vi "Autonomous Independent.vi"() -> ()   [LabVIEW 2017]
doc: "This VI is called when autonomous begins, and will automatically be terminated when autonomous ends. You can carry out timed or sensor driven robot movement independently without needing to return to the caller."
uses:
  <vilib>/Rock Robotics/WPI/Utilities/WPI_GetSetVariantRefNum.vi
  <vilib>/Rock Robotics/Network Tables/NT Read String.vi
  <vilib>/Rock Robotics/Network Tables/NT Read Number.vi
  <vilib>/Rock Robotics/Network Tables/NT Read Boolean.vi
  <vilib>/Rock Robotics/WPI/RobotDrive/WPI_RobotDriveArcadeDrive_Standard(NoSaturation).vi
  <vilib>/Rock Robotics/Network Tables/NT Write Numeric Array.vi
panel:
  in  "1 switch":T1(array[cluster])=[{"Movement"="Pause", "Delay (sec)"=1.0, "X Joystick Value"=0.0, "Y Joystick Value"=0.0}, {"Movement"="Forward 90 in", "Delay (sec)"=4.5, "X Joystick Value"=0.0, "Y Joystick Value"=0.5}, {"Movement"="Puase", "Delay (sec)"=1.0, "X Joystick Value"=0.0, "Y Joystick Value"=0.0}, {"Movement"="Slow Turn 90", "Delay (sec)"=0.55, "X Joystick Value"=0.7, "Y Joystick Value"=0.0}, {"Movement"="Pause", "Delay (sec)"=1.0, "X Joystick Value"=0.0, "Y Joystick Value"=0.0}, {"Movement"="Jolt", "Delay (sec)"=0.3, "X Joystick Value"=0.0, "Y Joystick Value"=1.0}, {"Movement"="Pause", "Delay (sec)"=1.0, "X Joystick Value"=0.0, "Y Joystick Value"=0.0}]
  in  "3 Switch":T1(array[cluster])=[{"Movement"="Pause", "Delay (sec)"=1.0, "X Joystick Value"=0.0, "Y Joystick Value"=0.0}, {"Movement"="Forward 90 in", "Delay (sec)"=4.5, "X Joystick Value"=0.0, "Y Joystick Value"=0.5}, {"Movement"="Puase", "Delay (sec)"=1.0, "X Joystick Value"=0.0, "Y Joystick Value"=0.0}, {"Movement"="slow turn 90", "Delay (sec)"=0.55, "X Joystick Value"=-0.7, "Y Joystick Value"=0.0}, {"Movement"="Pause", "Delay (sec)"=1.0, "X Joystick Value"=0.0, "Y Joystick Value"=0.0}, {"Movement"="Jolt", "Delay (sec)"=0.3, "X Joystick Value"=0.0, "Y Joystick Value"=1.0}, {"Movement"="Pause", "Delay (sec)"=1.0, "X Joystick Value"=0.0, "Y Joystick Value"=0.0}]
  in  "2 line 2":T1(array[cluster])=[{"Movement"="Pause", "Delay (sec)"=1.0, "X Joystick Value"=0.0, "Y Joystick Value"=0.0}, {"Movement"="Forward 90 in", "Delay (sec)"=4.5, "X Joystick Value"=0.0, "Y Joystick Value"=0.5}, {"Movement"="Puase", "Delay (sec)"=1.0, "X Joystick Value"=0.0, "Y Joystick Value"=0.0}, {"Movement"="Forward 60\nForward 60 in", "Delay (sec)"=1.0, "X Joystick Value"=0.0, "Y Joystick Value"=0.0}, {"Movement"="Forward 90 in", "Delay (sec)"=1.0, "X Joystick Value"=0.0, "Y Joystick Value"=0.0}, {"Movement"="Forward 90 in", "Delay (sec)"=1.0, "X Joystick Value"=0.0, "Y Joystick Value"=0.0}]
  in  "2 line 1":T1(array[cluster])=[{"Movement"="Pause", "Delay (sec)"=1.0, "X Joystick Value"=0.0, "Y Joystick Value"=0.0}, {"Movement"="Forward 90 in", "Delay (sec)"=4.5, "X Joystick Value"=0.0, "Y Joystick Value"=0.5}, {"Movement"="Puase", "Delay (sec)"=1.0, "X Joystick Value"=0.0, "Y Joystick Value"=0.0}, {"Movement"="Pause\nForward 60 in", "Delay (sec)"=1.0, "X Joystick Value"=0.0, "Y Joystick Value"=0.0}, {"Movement"="Pause", "Delay (sec)"=1.0, "X Joystick Value"=0.0, "Y Joystick Value"=0.0}, {"Movement"="Pause", "Delay (sec)"=1.0, "X Joystick Value"=0.0, "Y Joystick Value"=0.0}]
  in  "3 line":T1(array[cluster])=[{"Movement"="Pause", "Delay (sec)"=0.0, "X Joystick Value"=0.0, "Y Joystick Value"=0.0}, {"Movement"="Forward 90 in", "Delay (sec)"=4.5, "X Joystick Value"=0.0, "Y Joystick Value"=0.5}, {"Movement"="Puase", "Delay (sec)"=1.0, "X Joystick Value"=0.0, "Y Joystick Value"=0.0}, {"Movement"="Back ", "Delay (sec)"=1.0, "X Joystick Value"=0.0, "Y Joystick Value"=0.0}, {"Movement"="Forward 90 in", "Delay (sec)"=1.0, "X Joystick Value"=0.0, "Y Joystick Value"=0.0}, {"Movement"="Forward 90 in", "Delay (sec)"=1.0, "X Joystick Value"=0.0, "Y Joystick Value"=0.0}]
  in  "1 Line":T1(array[cluster])=[{"Movement"="Pause", "Delay (sec)"=1.0, "X Joystick Value"=0.0, "Y Joystick Value"=0.0}, {"Movement"="Forward 90 in", "Delay (sec)"=4.5, "X Joystick Value"=0.0, "Y Joystick Value"=0.5}, {"Movement"="Puase", "Delay (sec)"=1.0, "X Joystick Value"=0.0, "Y Joystick Value"=0.0}, {"Movement"="back 60\nForward 60 in", "Delay (sec)"=1.0, "X Joystick Value"=0.0, "Y Joystick Value"=0.0}, {"Movement"="Forward 90 in", "Delay (sec)"=1.0, "X Joystick Value"=0.0, "Y Joystick Value"=0.0}, {"Movement"="Forward 90 in", "Delay (sec)"=1.0, "X Joystick Value"=0.0, "Y Joystick Value"=0.0}]
  in  "Auto Main 2":T1(array[cluster])=[{"Movement"="Pause", "Delay (sec)"=1.0, "X Joystick Value"=0.0, "Y Joystick Value"=0.0}, {"Movement"="Forward 90 in", "Delay (sec)"=2.2, "X Joystick Value"=0.0, "Y Joystick Value"=0.7}, {"Movement"="Puase", "Delay (sec)"=1.0, "X Joystick Value"=0.0, "Y Joystick Value"=0.0}, {"Movement"="Forward 60\nForward 60 in", "Delay (sec)"=1.0, "X Joystick Value"=0.0, "Y Joystick Value"=0.0}, {"Movement"="Forward 90 in", "Delay (sec)"=1.0, "X Joystick Value"=0.0, "Y Joystick Value"=0.0}, {"Movement"="Forward 90 in", "Delay (sec)"=1.0, "X Joystick Value"=0.0, "Y Joystick Value"=0.0}]
  out "Current Movement, for debugging":T2 {"Y Joystick Value" scale=1.0..-1.0; "X Joystick Value" scale=-1.0..1.0}
  in  "Array of robot movements":T3(array[cluster])=[{"X Joystick Value"=0.39393939393939403, "Y Joystick Value"=0.0, "Delay (sec)"=1.0, "Movement Name"="turn"}, {"X Joystick Value"=-0.3737373737373737, "Y Joystick Value"=0.0, "Delay (sec)"=1.0, "Movement Name"="turn back"}] {"Y Joystick Value" scale=1.0..-1.0; "X Joystick Value" scale=-1.0..1.0}
  # "Be sure to right-click and choose Data Operations>>Make Current Value default if you want to save the array values with the VI"
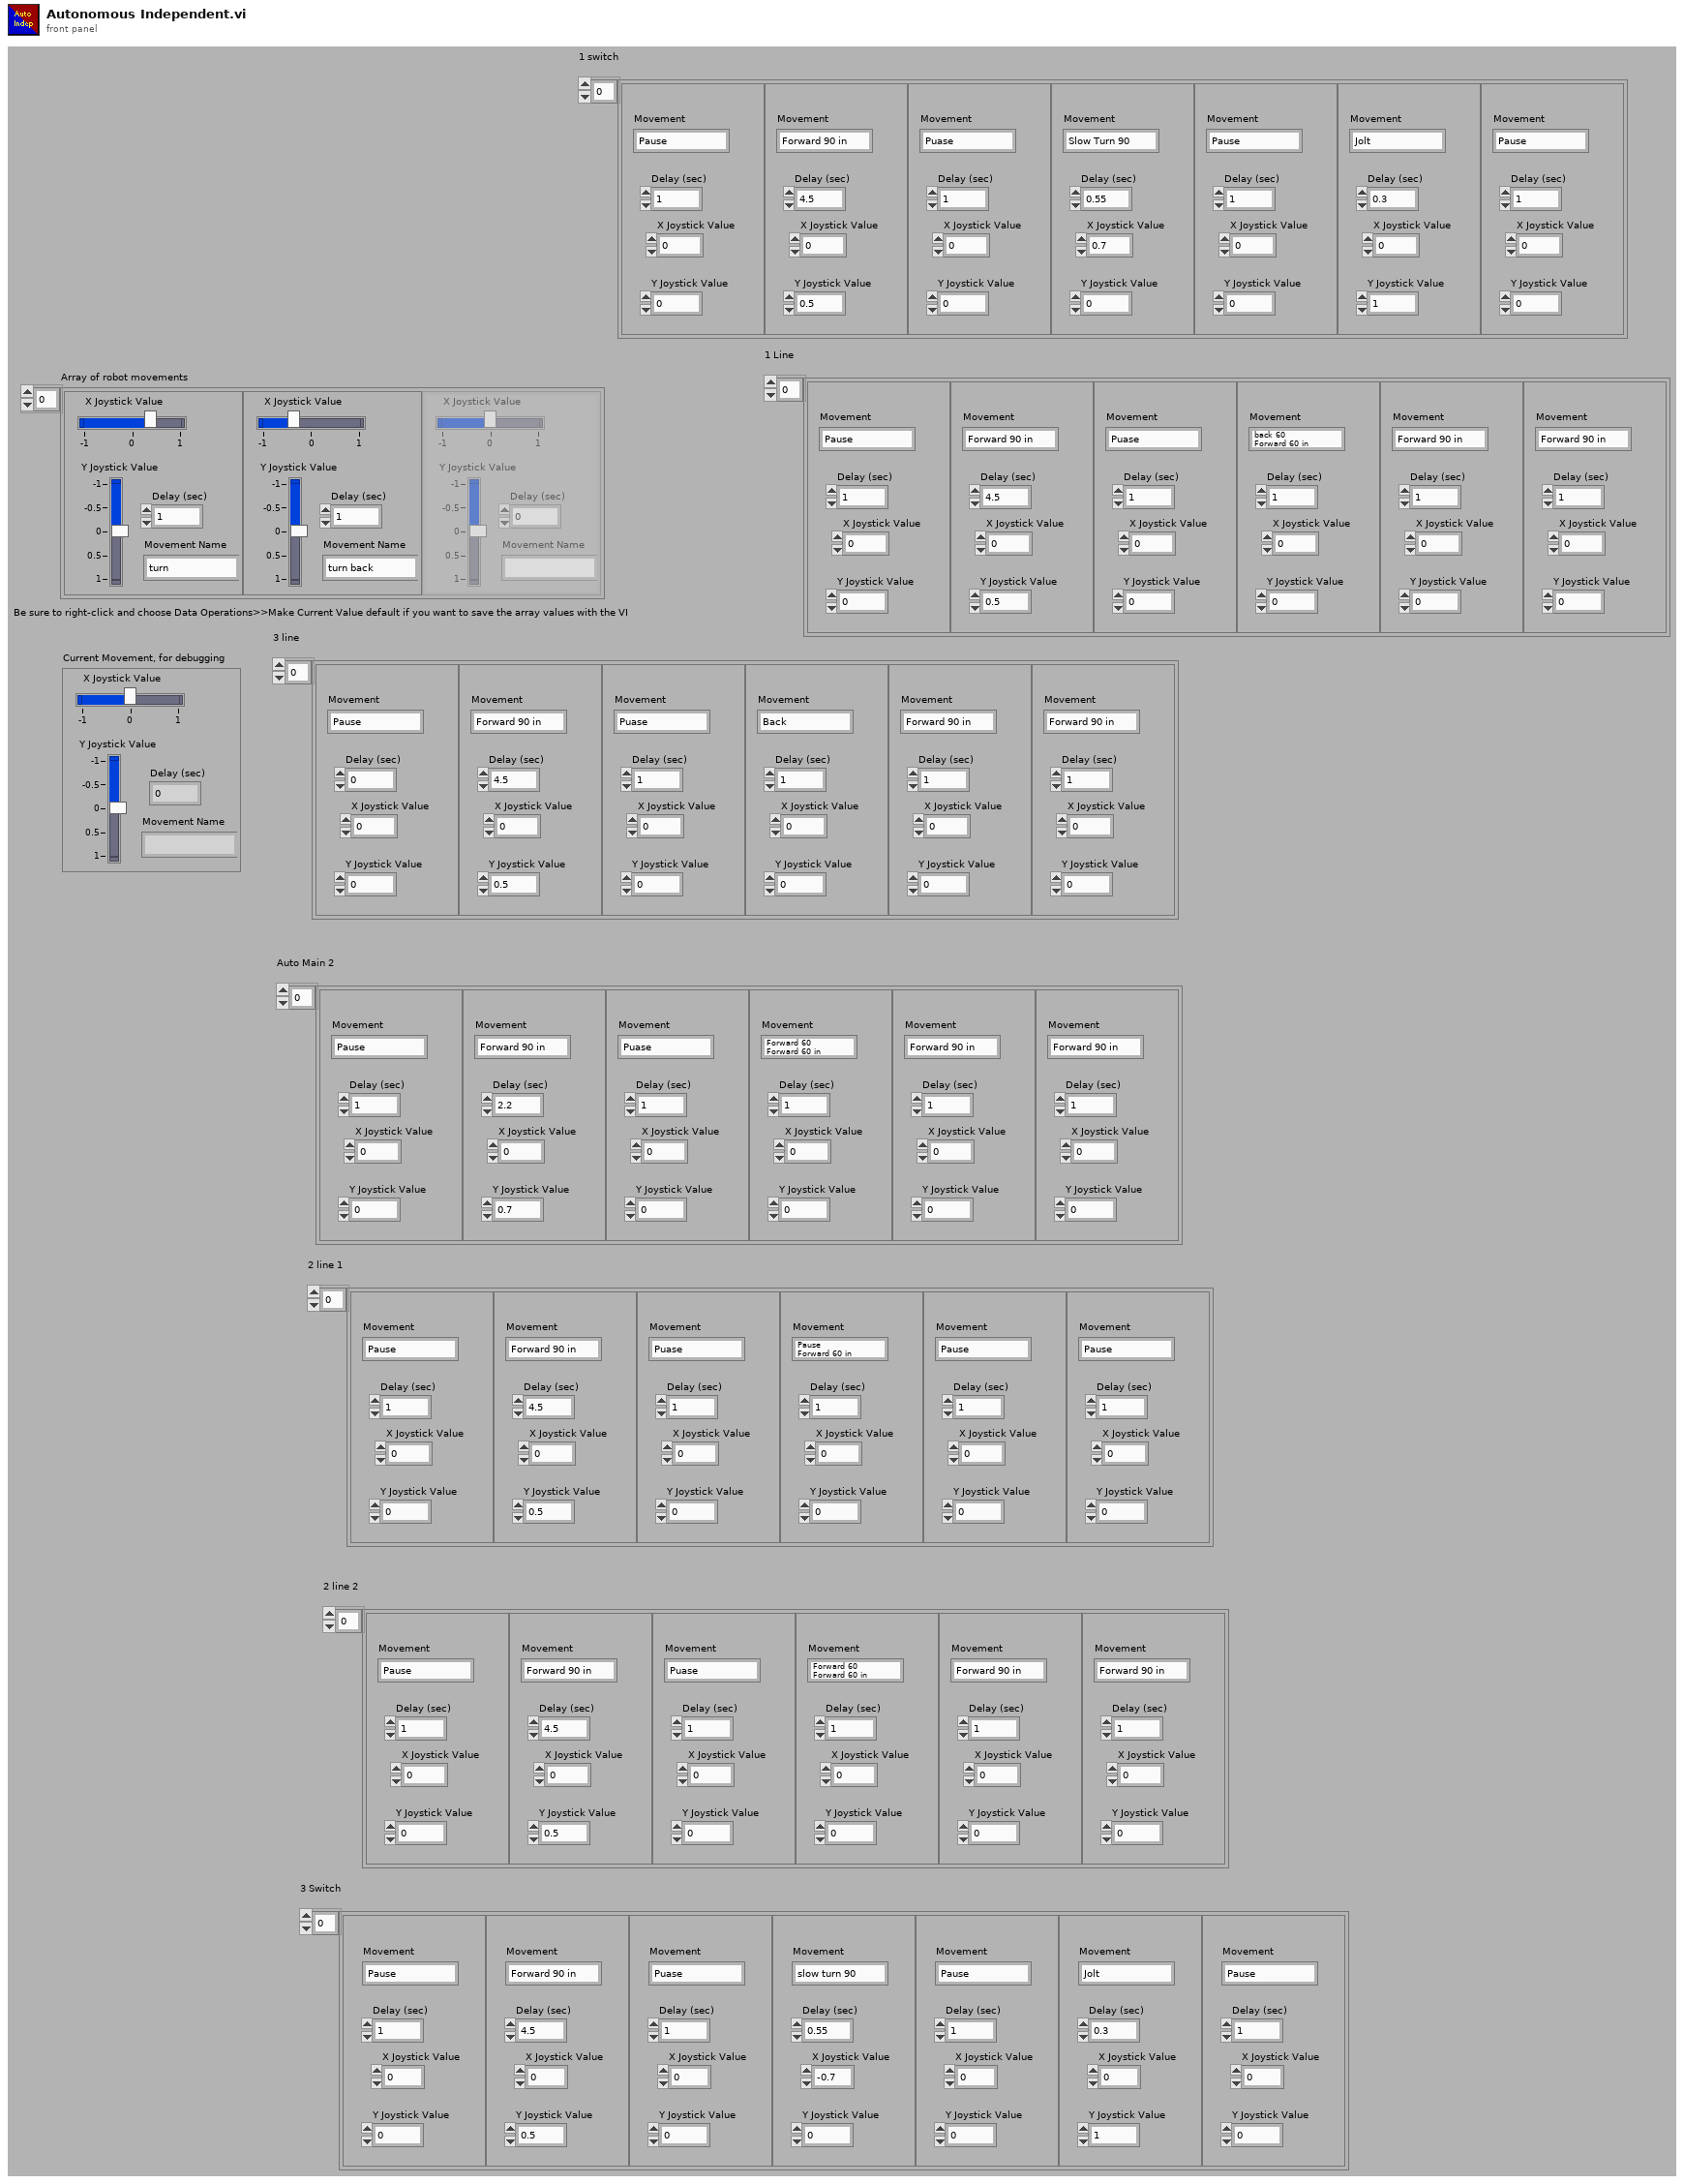
[diagram p1: front panel]
types:
  T1 = cluster{"Movement":string, "Delay (sec)":dbl, "X Joystick Value":dbl, "Y Joystick Value":dbl}[]
  T2 = cluster{"X Joystick Value":dbl, "Y Joystick Value":dbl, "Delay (sec)":dbl, "Movement Name":string}
  T3 = cluster{"X Joystick Value":dbl, "Y Joystick Value":dbl, "Delay (sec)":dbl, "Movement Name":string}[]
  T4 = typedef "WPI_JoystickDevRef.ctl" = cluster{"Device":T5}
  T5 = typedef "WPI_JoystickDeviceEnum.ctl" = enum16{"USB 0", "USB 1", "USB 2", "USB 3", "USB 4", "USB 5"}
  T6 = typedef "WPI_RobotDriveDevRef.ctl" = cluster{"DevStatus":errorcluster, "Motors[]":T7[], "Square Inputs":bool, "Max Output":dbl}
  T7 = typedef "WPI_MotorControlDeviceRef.ctl" = cluster{"DeviceStatus":errorcluster, "Type":T8, "PWM":cluster{"PWM Channel":T9, "DeadBand":T10}, "CAN":cluster{"Device Number":u8, "SetOutput VI Ref":variant, "GetOutput VI Ref":variant, "Enable VI Ref":variant, "Disable VI Ref":variant, "Data":variant}, "Invert":bool, "DIO PWM":cluster{"PWM \"Enable\" Channel":T9, "DIOChannel":T11, "PWM Rate":dbl}}
  T8 = typedef "WPI_MotorControlType.ctl" = enum16{"PWM", "CAN", "DIO PWM"}
  T9 = typedef "FPGA_DIOPWMChannel.ctl" = enum8{"PWM 0", "PWM 1", "PWM 2", "PWM 3", "PWM 4", "PWM 5", "PWM 6", "PWM 7", "PWM 8", "PWM 9", "PWM MXP 0", "PWM MXP 1", "PWM MXP 2", "PWM MXP 3", "PWM MXP 4", "PWM MXP 5", "PWM MXP 6", "PWM MXP 7", "PWM MXP 8", "PWM MXP 9", "Invalid"}
  T10 = typedef "WPI_PWMDeadband.ctl" = cluster{"Name":string, "maxPositivePwm":i32, "minPositivePwm":i32, "centerPwm":i32, "maxNegativePwm":i32, "minNegativePwm":i32, "angularRange":u16}
  T11 = typedef "FPGA_DIOChannel.ctl" = enum8{"DIO 0", "DIO 1", "DIO 2", "DIO 3", "DIO 4", "DIO 5", "DIO 6", "DIO 7", "DIO 8", "DIO 9", "DIO MXP 0", "DIO MXP 1", "DIO MXP 2", "DIO MXP 3", "DIO MXP 4", "DIO MXP 5", "DIO MXP 6", "DIO MXP 7", "DIO MXP 8", "DIO MXP 9", "DIO MXP 10", "DIO MXP 11", "DIO MXP 12", "DIO MXP 13", "DIO MXP 14", "DIO MXP 15", "SPI Port CS1", "SPI Port CS2", "SPI Port CS3", "SPI Port MISO", "SPI Port MOSI", "Invalid"}
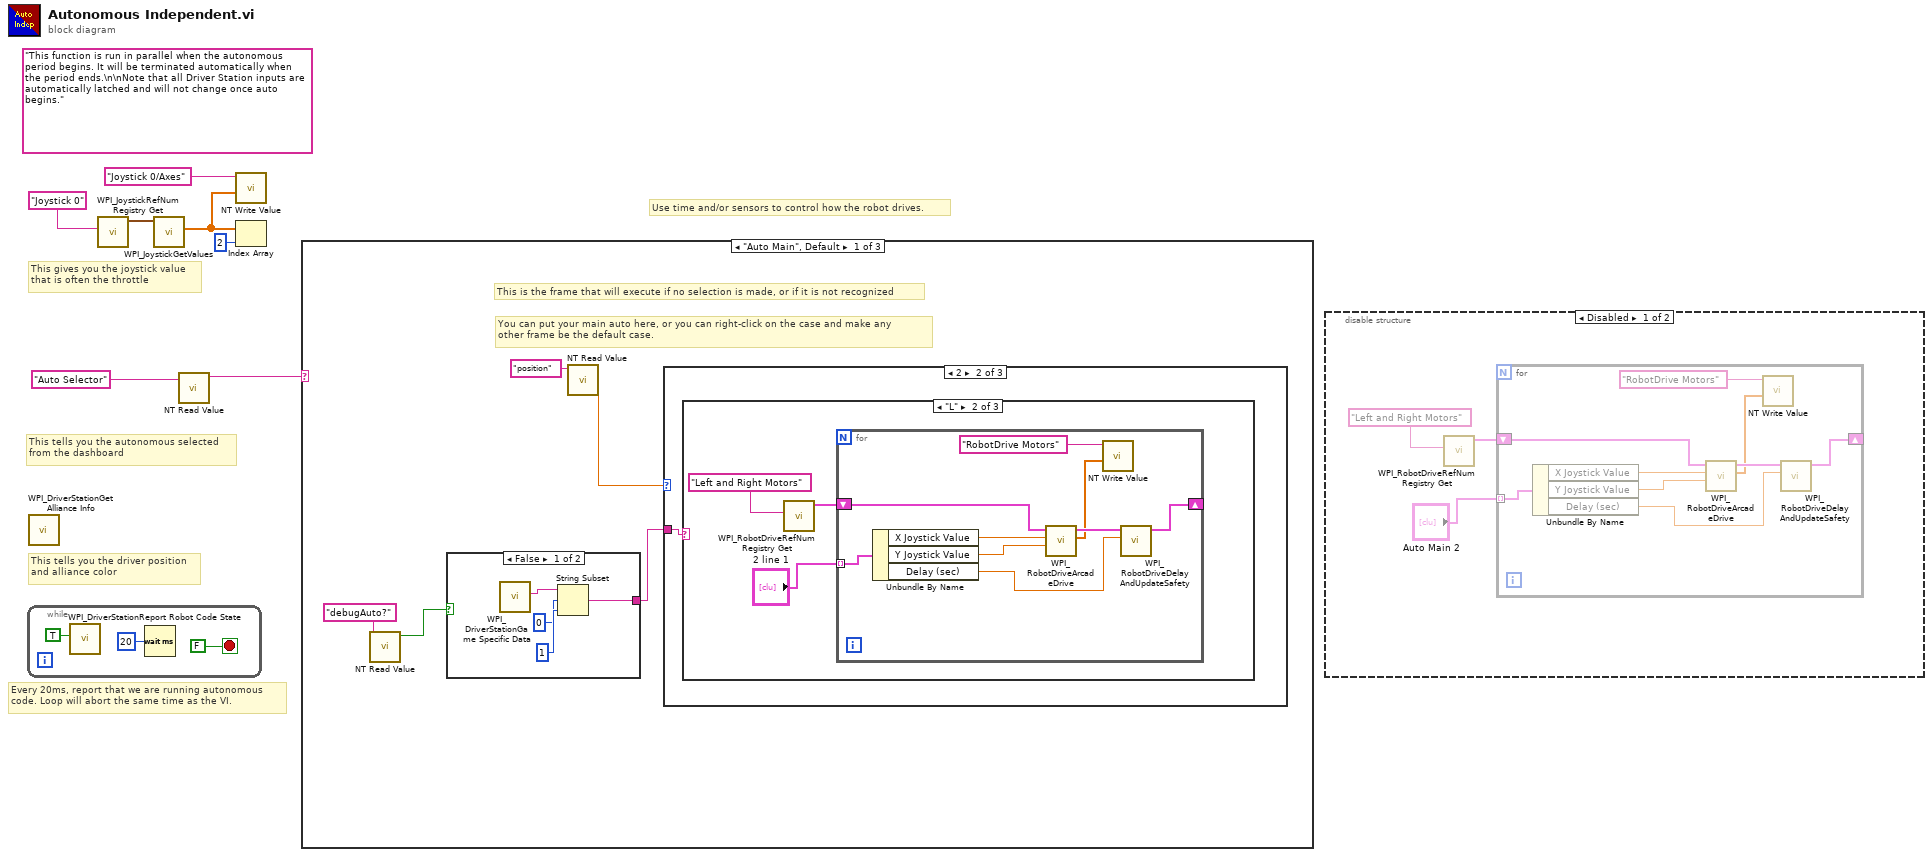
[diagram p0: block diagram]
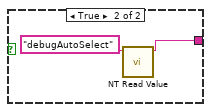
[diagram p3: hidden frame]
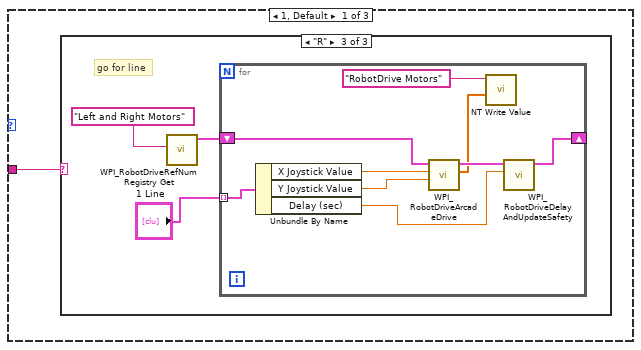
[diagram p4: hidden frame]
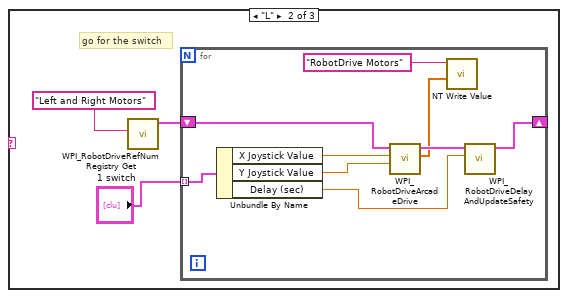
[diagram p6: hidden frame]
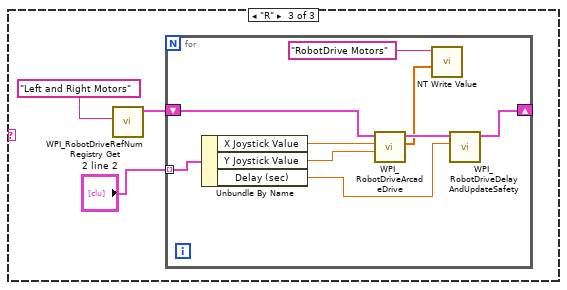
[diagram p8: hidden frame]
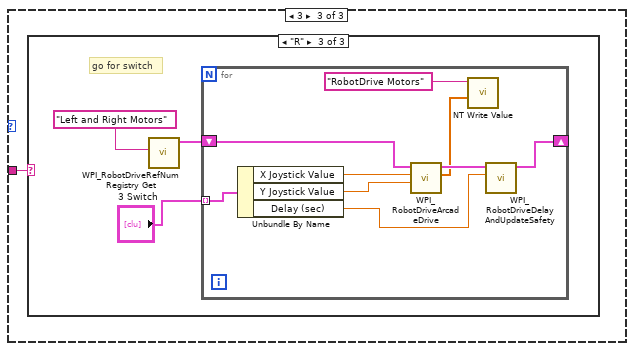
[diagram p9: hidden frame]
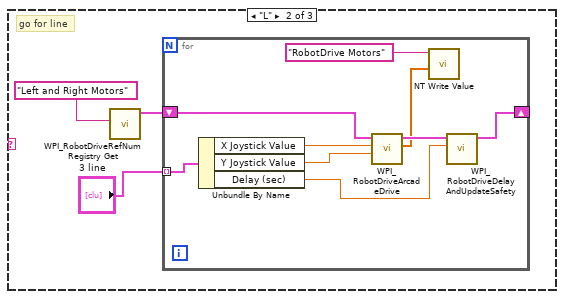
[diagram p11: hidden frame]
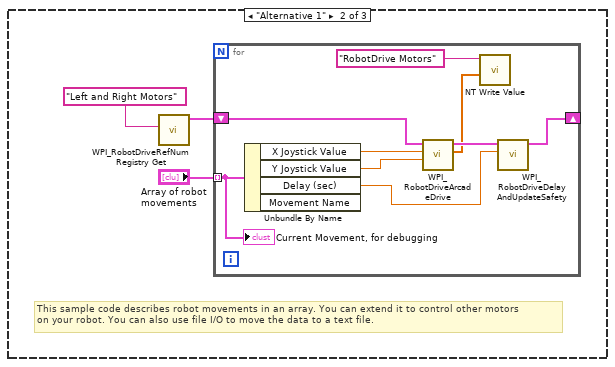
[diagram p12: hidden frame]
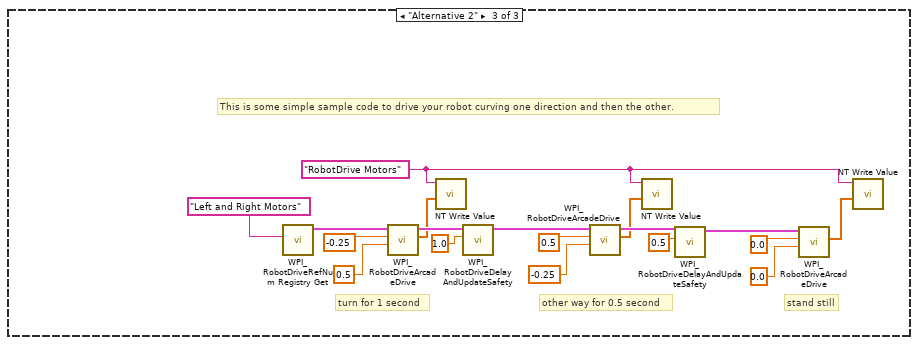
[diagram p13: hidden frame]
diagram:
  (unwired) "This function is run in parallel when the autonomous period begins. It will be terminated automatically when the period ends.\n\nNote that all Driver Station inputs are automatically latched and will not change once auto begins."
  # "This tells you the autonomous selected\nfrom the dashboard"
  # "Every 20ms, report that we are running autonomous\ncode. Loop will abort the same time as the VI."
  # "This gives you the joystick value\nthat is often the throttle"
  # "Use time and/or sensors to control how the robot drives."
  # "This tells you the driver position\nand alliance color"
  n1 = while {
    stop <- FALSE stop-if-true
    n2 = call <vilib>:"WPI_DriverStationReport Robot Code State.vi"("Autonomous"=TRUE) -> ()  [unwired: 10 in, 1 out]
    n3 = Wait (ms)(milliseconds to wait=u32 20) -> ()  [unwired: 1 out]
  }
  n4 = call <vilib>:"WPI_DriverStationGet Alliance Info.vi"() -> ()  [unwired: 12 out]
  n5 = call <vilib>:"WPI_JoystickRefNum Registry Get.vi"("refnum name"="Joystick 0") -> ("JoystickDevRef"=w6:T4)  [unwired: 1 in, 9 out]
  n6 = call <vilib>:"WPI_JoystickGetValues.vi"("JoystickDevRef"=w6) -> ("Axes"=w2:dbl[])  [unwired: 6 in, 4 out]
  n7 = call-poly <vilib>:"NT Read Value.vi"("Name"="Auto Selector") -> ("String"=w3:string)  [unwired: 9 in, 1 out]
  n8 = call-poly <vilib>:"NT Write Value.vi"("Numeric Array"=w2, "Name"="Joystick 0/Axes") -> ()  [unwired: 9 in, 1 out]
  n9 = Index Array(array=w2, index=2) -> ()  [unwired: 1 out]
  n10 = case shown="\"Auto Main\", Default" w3 {
    frame "Auto Main", Default {
      # "You can put your main auto here, or you can right-click on the case and make any\nother frame be the default case."
      # "This is the frame that will execute if no selection is made, or if it is not recognized"
      n11 = call-poly <vilib>:"NT Read Value.vi"("Name"="debugAuto?") -> ("Boolean"=w12:bool)  [unwired: 9 in, 1 out]
      n12 = case shown="False" w12 {
        tunnel: [w16 w20] -> w15
        frame False {
          n13 = call <vilib>:"WPI_DriverStationGame Specific Data.vi"() -> ("Game Specific Data"=w19:string)  [unwired: 11 in]
          n14 = String Subset(string=w19, offset (0)=0, length (rest)=1 ("length (rest)")) -> (substring=w16:string)
        }
        frame True {
          n15 = call-poly <vilib>:"NT Read Value.vi"("Name"="debugAutoSelect") -> ("String"=w20:string)  [unwired: 9 in, 1 out]
        }
      }
      n16 = call-poly <vilib>:"NT Read Value.vi"("Name"="position") -> ("Numeric"=w13:dbl)  [unwired: 9 in, 1 out]
      n17 = case shown="2" w13 {
        tunnel: w15 -> [w22 w47 w72]
        frame 1, Default {
          n18 = case shown="\"R\"" w22 {
            frame Default {
            }
            frame "L" {
              # "go for the switch"
              n19 = call <vilib>:"WPI_RobotDriveRefNum Registry Get.vi"("refnum name"="Left and Right Motors") -> ("RobotDriveDevRef"=w24:T6)  [unwired: 1 in, 9 out]
              n20 = for {
                shift-right: [w32] -> _
                shift-left: w24 -> [w33]
                tunnel: "1 switch" -> [w28] mode=indexing
                n21 = Unbundle By Name(w28) -> ("X Joystick Value"=w31:dbl, "Y Joystick Value"=w30:dbl, "Delay (sec)"=w29:dbl)
                n22 = call-poly <vilib>:"WPI_RobotDriveArcadeDrive.vi"("Y axis value"=w30, "X axis value"=w31, "RobotDriveDevRef"=w33) -> ("Motor Values"=w26:dbl[], "RobotDriveDevRef"=w34:T6)  [unwired: 1 in, 6 out]
                n23 = call-poly <vilib>:"NT Write Value.vi"("Numeric Array"=w26, "Name"="RobotDrive Motors") -> ()  [unwired: 9 in, 1 out]
                n24 = call <vilib>:"WPI_RobotDriveDelayAndUpdateSafety.vi"("Delay (s)"=w29, "RobotDriveDevRef"=w34) -> ("RobotDriveDevRef 2"=w32:T6)  [unwired: 8 in, 1 out]
              }
            }
            frame "R" {
              # "go for line"
              n25 = call <vilib>:"WPI_RobotDriveRefNum Registry Get.vi"("refnum name"="Left and Right Motors") -> ("RobotDriveDevRef"=w36:T6)  [unwired: 1 in, 9 out]
              n26 = for {
                shift-right: [w44] -> _
                shift-left: w36 -> [w45]
                tunnel: "1 Line" -> [w40] mode=indexing
                n27 = Unbundle By Name(w40) -> ("X Joystick Value"=w43:dbl, "Y Joystick Value"=w42:dbl, "Delay (sec)"=w41:dbl)
                n28 = call-poly <vilib>:"WPI_RobotDriveArcadeDrive.vi"("Y axis value"=w42, "X axis value"=w43, "RobotDriveDevRef"=w45) -> ("Motor Values"=w38:dbl[], "RobotDriveDevRef"=w46:T6)  [unwired: 1 in, 6 out]
                n29 = call-poly <vilib>:"NT Write Value.vi"("Numeric Array"=w38, "Name"="RobotDrive Motors") -> ()  [unwired: 9 in, 1 out]
                n30 = call <vilib>:"WPI_RobotDriveDelayAndUpdateSafety.vi"("Delay (s)"=w41, "RobotDriveDevRef"=w46) -> ("RobotDriveDevRef 2"=w44:T6)  [unwired: 8 in, 1 out]
              }
            }
          }
        }
        frame 2 {
          n31 = case shown="\"L\"" w47 {
            frame Default {
            }
            frame "L" {
              n32 = call <vilib>:"WPI_RobotDriveRefNum Registry Get.vi"("refnum name"="Left and Right Motors") -> ("RobotDriveDevRef"=w49:T6)  [unwired: 1 in, 9 out]
              n33 = for {
                shift-right: [w57] -> _
                shift-left: w49 -> [w58]
                tunnel: "2 line 1" -> [w53] mode=indexing
                n34 = Unbundle By Name(w53) -> ("X Joystick Value"=w56:dbl, "Y Joystick Value"=w55:dbl, "Delay (sec)"=w54:dbl)
                n35 = call-poly <vilib>:"WPI_RobotDriveArcadeDrive.vi"("Y axis value"=w55, "X axis value"=w56, "RobotDriveDevRef"=w58) -> ("Motor Values"=w51:dbl[], "RobotDriveDevRef"=w59:T6)  [unwired: 1 in, 6 out]
                n36 = call-poly <vilib>:"NT Write Value.vi"("Numeric Array"=w51, "Name"="RobotDrive Motors") -> ()  [unwired: 9 in, 1 out]
                n37 = call <vilib>:"WPI_RobotDriveDelayAndUpdateSafety.vi"("Delay (s)"=w54, "RobotDriveDevRef"=w59) -> ("RobotDriveDevRef 2"=w57:T6)  [unwired: 8 in, 1 out]
              }
            }
            frame "R" {
              n38 = call <vilib>:"WPI_RobotDriveRefNum Registry Get.vi"("refnum name"="Left and Right Motors") -> ("RobotDriveDevRef"=w61:T6)  [unwired: 1 in, 9 out]
              n39 = for {
                shift-right: [w69] -> _
                shift-left: w61 -> [w70]
                tunnel: "2 line 2" -> [w65] mode=indexing
                n40 = Unbundle By Name(w65) -> ("X Joystick Value"=w68:dbl, "Y Joystick Value"=w67:dbl, "Delay (sec)"=w66:dbl)
                n41 = call-poly <vilib>:"WPI_RobotDriveArcadeDrive.vi"("Y axis value"=w67, "X axis value"=w68, "RobotDriveDevRef"=w70) -> ("Motor Values"=w63:dbl[], "RobotDriveDevRef"=w71:T6)  [unwired: 1 in, 6 out]
                n42 = call-poly <vilib>:"NT Write Value.vi"("Numeric Array"=w63, "Name"="RobotDrive Motors") -> ()  [unwired: 9 in, 1 out]
                n43 = call <vilib>:"WPI_RobotDriveDelayAndUpdateSafety.vi"("Delay (s)"=w66, "RobotDriveDevRef"=w71) -> ("RobotDriveDevRef 2"=w69:T6)  [unwired: 8 in, 1 out]
              }
            }
          }
        }
        frame 3 {
          n44 = case shown="\"R\"" w72 {
            frame Default {
            }
            frame "L" {
              # "go for line"
              n45 = call <vilib>:"WPI_RobotDriveRefNum Registry Get.vi"("refnum name"="Left and Right Motors") -> ("RobotDriveDevRef"=w74:T6)  [unwired: 1 in, 9 out]
              n46 = for {
                shift-right: [w82] -> _
                shift-left: w74 -> [w83]
                tunnel: "3 line" -> [w78] mode=indexing
                n47 = Unbundle By Name(w78) -> ("X Joystick Value"=w81:dbl, "Y Joystick Value"=w80:dbl, "Delay (sec)"=w79:dbl)
                n48 = call-poly <vilib>:"WPI_RobotDriveArcadeDrive.vi"("Y axis value"=w80, "X axis value"=w81, "RobotDriveDevRef"=w83) -> ("Motor Values"=w76:dbl[], "RobotDriveDevRef"=w84:T6)  [unwired: 1 in, 6 out]
                n49 = call-poly <vilib>:"NT Write Value.vi"("Numeric Array"=w76, "Name"="RobotDrive Motors") -> ()  [unwired: 9 in, 1 out]
                n50 = call <vilib>:"WPI_RobotDriveDelayAndUpdateSafety.vi"("Delay (s)"=w79, "RobotDriveDevRef"=w84) -> ("RobotDriveDevRef 2"=w82:T6)  [unwired: 8 in, 1 out]
              }
            }
            frame "R" {
              # "go for switch"
              n51 = call <vilib>:"WPI_RobotDriveRefNum Registry Get.vi"("refnum name"="Left and Right Motors") -> ("RobotDriveDevRef"=w86:T6)  [unwired: 1 in, 9 out]
              n52 = for {
                shift-right: [w94] -> _
                shift-left: w86 -> [w95]
                tunnel: "3 Switch" -> [w90] mode=indexing
                n53 = Unbundle By Name(w90) -> ("X Joystick Value"=w93:dbl, "Y Joystick Value"=w92:dbl, "Delay (sec)"=w91:dbl)
                n54 = call-poly <vilib>:"WPI_RobotDriveArcadeDrive.vi"("Y axis value"=w92, "X axis value"=w93, "RobotDriveDevRef"=w95) -> ("Motor Values"=w88:dbl[], "RobotDriveDevRef"=w96:T6)  [unwired: 1 in, 6 out]
                n55 = call-poly <vilib>:"NT Write Value.vi"("Numeric Array"=w88, "Name"="RobotDrive Motors") -> ()  [unwired: 9 in, 1 out]
                n56 = call <vilib>:"WPI_RobotDriveDelayAndUpdateSafety.vi"("Delay (s)"=w91, "RobotDriveDevRef"=w96) -> ("RobotDriveDevRef 2"=w94:T6)  [unwired: 8 in, 1 out]
              }
            }
          }
        }
      }
    }
    frame "Alternative 1" {
      # "This sample code describes robot movements in an array. You can extend it to control other motors\non your robot. You can also use file I/O to move the data to a text file."
      n57 = call <vilib>:"WPI_RobotDriveRefNum Registry Get.vi"("refnum name"="Left and Right Motors") -> ("RobotDriveDevRef"=w98:T6)  [unwired: 1 in, 9 out]
      n58 = for {
        shift-right: [w106] -> _
        shift-left: w98 -> [w107]
        tunnel: "Array of robot movements" -> [w102] mode=indexing
        n59 = Unbundle By Name(w102) -> ("X Joystick Value"=w105:dbl, "Y Joystick Value"=w104:dbl, "Delay (sec)"=w103:dbl)  [unwired: 1 out]
        n60 = call-poly <vilib>:"WPI_RobotDriveArcadeDrive.vi"("Y axis value"=w104, "X axis value"=w105, "RobotDriveDevRef"=w107) -> ("Motor Values"=w100:dbl[], "RobotDriveDevRef"=w108:T6)  [unwired: 1 in, 6 out]
        n61 = call-poly <vilib>:"NT Write Value.vi"("Numeric Array"=w100, "Name"="RobotDrive Motors") -> ()  [unwired: 9 in, 1 out]
        n62 = call <vilib>:"WPI_RobotDriveDelayAndUpdateSafety.vi"("Delay (s)"=w103, "RobotDriveDevRef"=w108) -> ("RobotDriveDevRef 2"=w106:T6)  [unwired: 8 in, 1 out]
        "Current Movement, for debugging" <- w102
      }
    }
    frame "Alternative 2" {
      w110 = "RobotDrive Motors" ("Name")
      # "This is some simple sample code to drive your robot curving one direction and then the other."
      # "stand still"
      # "other way for 0.5 second"
      # "turn for 1 second"
      n63 = call <vilib>:"WPI_RobotDriveRefNum Registry Get.vi"("refnum name"="Left and Right Motors") -> ("RobotDriveDevRef"=w126:T6)  [unwired: 1 in, 9 out]
      n64 = call-poly <vilib>:"WPI_RobotDriveArcadeDrive.vi"("Y axis value"=0.5 ("X axis value"), "X axis value"=-0.25, "RobotDriveDevRef"=w126) -> ("Motor Values"=w109:dbl[], "RobotDriveDevRef"=w119:T6)  [unwired: 1 in, 6 out]
      n65 = call-poly <vilib>:"NT Write Value.vi"("Numeric Array"=w109, "Name"=w110) -> ()  [unwired: 9 in, 1 out]
      n66 = call <vilib>:"WPI_RobotDriveDelayAndUpdateSafety.vi"("Delay (s)"=1.0, "RobotDriveDevRef"=w119) -> ("RobotDriveDevRef 2"=w120:T6)  [unwired: 8 in, 1 out]
      n67 = call-poly <vilib>:"WPI_RobotDriveArcadeDrive.vi"("Y axis value"=-0.25 ("X axis value"), "X axis value"=0.5, "RobotDriveDevRef"=w120) -> ("Motor Values"=w111:dbl[], "RobotDriveDevRef"=w121:T6)  [unwired: 1 in, 6 out]
      n68 = call-poly <vilib>:"NT Write Value.vi"("Numeric Array"=w111, "Name"=w110) -> ()  [unwired: 9 in, 1 out]
      n69 = call <vilib>:"WPI_RobotDriveDelayAndUpdateSafety.vi"("Delay (s)"=0.5, "RobotDriveDevRef"=w121) -> ("RobotDriveDevRef 2"=w122:T6)  [unwired: 8 in, 1 out]
      n70 = call-poly <vilib>:"WPI_RobotDriveArcadeDrive.vi"("Y axis value"=0.0 ("X axis value"), "X axis value"=0.0, "RobotDriveDevRef"=w122) -> ("Motor Values"=w112:dbl[])  [unwired: 1 in, 7 out]
      n71 = call-poly <vilib>:"NT Write Value.vi"("Numeric Array"=w112, "Name"=w110) -> ()  [unwired: 9 in, 1 out]
    }
  }
  n72 = disable-structure shown="Disabled" {
    frame Disabled {
      n73 = call <vilib>:"WPI_RobotDriveRefNum Registry Get.vi"("refnum name"="Left and Right Motors") -> ("RobotDriveDevRef"=w128:T6)  [unwired: 1 in, 9 out]
      n74 = for {
        shift-right: [w136] -> _
        shift-left: w128 -> [w137]
        tunnel: "Auto Main 2" -> [w132] mode=indexing
        n75 = Unbundle By Name(w132) -> ("X Joystick Value"=w135:dbl, "Y Joystick Value"=w134:dbl, "Delay (sec)"=w133:dbl)
        n76 = call-poly <vilib>:"WPI_RobotDriveArcadeDrive.vi"("Y axis value"=w134, "X axis value"=w135, "RobotDriveDevRef"=w137) -> ("Motor Values"=w130:dbl[], "RobotDriveDevRef"=w138:T6)  [unwired: 1 in, 6 out]
        n77 = call-poly <vilib>:"NT Write Value.vi"("Numeric Array"=w130, "Name"="RobotDrive Motors") -> ()  [unwired: 9 in, 1 out]
        n78 = call <vilib>:"WPI_RobotDriveDelayAndUpdateSafety.vi"("Delay (s)"=w133, "RobotDriveDevRef"=w138) -> ("RobotDriveDevRef 2"=w136:T6)  [unwired: 8 in, 1 out]
      }
    }
    frame Enabled {
    }
  }
